vi "Read Math.vi"(0 "VISA resource name":refnum<visa-resource-name>, 5 "Buffer Name (\"\")":string, 7 "Channel List(\"\")":string, 9 "Clear (F: Disable)":bool, 11 "error in (no error)":errorcluster) -> (3 "Peak To Peak":dbl, 4 "VISA resource name out":refnum<visa-resource-name>, 6 "Average":dbl, 8 "Maximum":dbl, 10 "Minimum":dbl, 14 "Standard Deviation":dbl, 15 "error out":errorcluster)   [LabVIEW 2016, in "Keithley DMM6500 DAQ6500 Series.lvlib"]
doc: "Returns the math readings specified by the \"Buffer Name\""
uses:
  Keithley DMM6500 DAQ6500 Series.lvlib
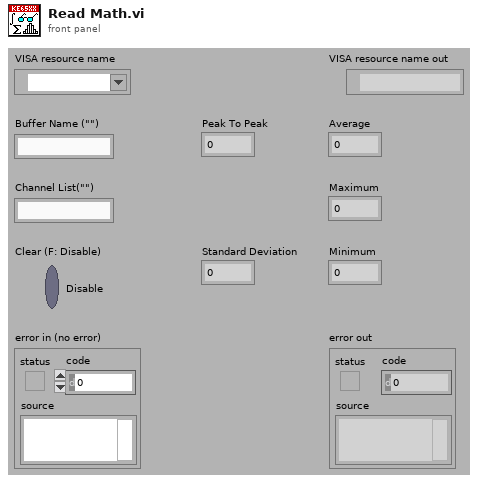
[diagram p1: front panel]
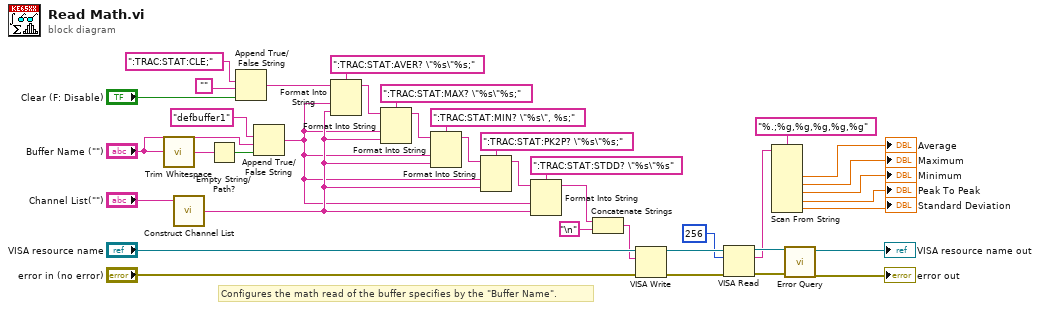
[diagram p0: block diagram]
diagram:
  # "Configures the math read of the buffer specifies by the \"Buffer Name\"."
  n1 = call <vilib>:"Trim Whitespace.vi"("string"="Buffer Name (\"\")") -> ("trimmed string"=w5:string)  [unwired: 1 in]
  n2 = call "Construct Channel List.vi"("Channel List"="Channel List(\"\")") -> ("Channel List String"=w18:string)  [unwired: 2 in]
  n3 = Empty String/Path?(string/path=w5) -> (empty?=w4:bool)
  n4 = Append True/False String(1:"Clear (F: Disable)", 2:"" ("Empty String Constant"), 3:":TRAC:STAT:CLE;") -> (0:w20:string)  [unwired: 1 in]
  n5 = Append True/False String(1:w4, 2:"Buffer Name (\"\")", 3:"defbuffer1" ("true string")) -> (0:w1:string)  [unwired: 1 in]
  n6 = Format Into String(format string=":TRAC:STAT:AVER? \"%s\"%s;", initial string=w20, w1, w18) -> (resulting string=w38:string)  [unwired: 1 in, 1 out]
  n7 = Format Into String(format string=":TRAC:STAT:MAX? \"%s\"%s;", initial string=w38, w1, w18) -> (resulting string=w36:string)  [unwired: 1 in, 1 out]
  n8 = Format Into String(format string=":TRAC:STAT:MIN? \"%s\", %s;", initial string=w36, w1, w18) -> (resulting string=w34:string)  [unwired: 1 in, 1 out]
  n9 = Format Into String(format string=":TRAC:STAT:PK2P? \"%s\"%s;", initial string=w34, w1, w18) -> (resulting string=w32:string)  [unwired: 1 in, 1 out]
  n10 = Format Into String(format string=":TRAC:STAT:STDD? \"%s\"%s", initial string=w32, w1, w18) -> (resulting string=w25:string)  [unwired: 1 in, 1 out]
  n11 = Concatenate Strings(w25, "\n" ("Line Feed Constant")) -> (w26:string)
  n12 = VISA Write(VISA resource name="VISA resource name", write buffer=w26, error in (no error)="error in (no error)") -> (VISA resource name out=w16:refnum<visa-resource-name>, error out=w15:errorcluster)  [unwired: 1 out]
  n13 = VISA Read(VISA resource name=w16, byte count=u32 256, error in (no error)=w15) -> (VISA resource name out=w17:refnum<visa-resource-name>, read buffer=w12:string, error out=w14:errorcluster)  [unwired: 1 out]
  n14 = Scan From String(format string="%.;%g,%g,%g,%g,%g", input string=w12) -> (output 1=→"Average":dbl, output 2=→"Maximum":dbl, output 3=→"Minimum":dbl, output 4=→"Peak To Peak":dbl, output 5=→"Standard Deviation":dbl)  [unwired: 7 in, 3 out]
  n15 = call "Error Query.vi"("error in (no error)"=w14, "VISA resource name"=w17) -> ("error out"=→"error out":errorcluster, "VISA resource name out"=→"VISA resource name out":refnum<visa-resource-name>)  [unwired: 6 in, 2 out]
